vi "HP4263B_CommandsGlobal.vi"() -> ()   [LabVIEW 2013, in "HP4263B.lvclass"]
uses:
  HP4263B.lvclass
panel:
  in  "HP 4263B GPIB Setup":T1={"Instrument name"="HP 4263B", "Instrument type"=1, "Command \"Initialise LCR\""=":sense:func:conc off;:sense:func %s;:calc1:form %s; :calc2:form %s;:source:frequency:cw  %d;:source:voltage %d MV;:trigger:source bus;:cal:cable %d;:sens:aver:count %d; :sense:average:state %s;", "Command \"OC Trim\""="", "Command \"LCR Readout\""=""} {"Instrument type" items=["Supply", "LCR"]}
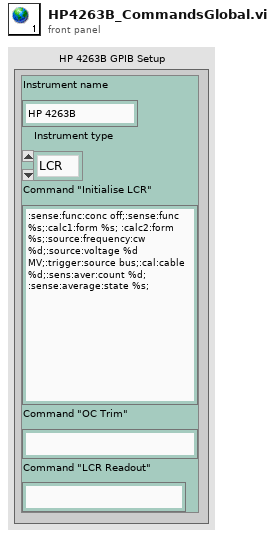
[diagram p1: front panel]
types:
  T1 = cluster{"Instrument name":string, "Instrument type":u16, "Command \"Initialise LCR\"":string, "Command \"OC Trim\"":string, "Command \"LCR Readout\"":string}
diagram:
